vi "练习3.2-连续改变输出频率.vi"() -> ()   [LabVIEW 2021]
panel:
  out "Waveform Graph":dynamicdata(graph)
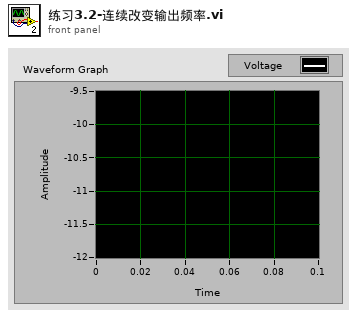
[diagram p1: front panel]
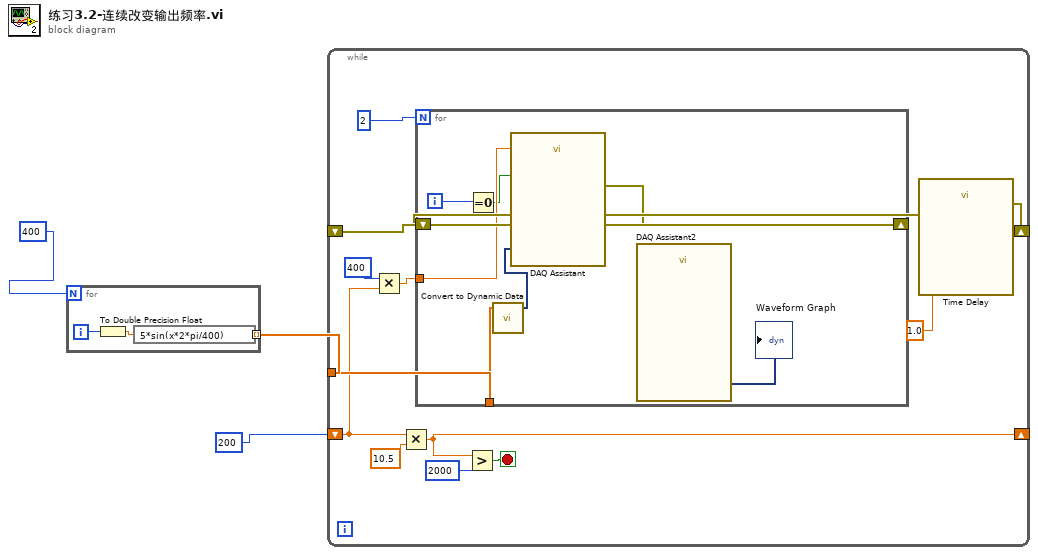
[diagram p0: block diagram]
diagram:
  n1 = for {
    N: 400 -> [_]
    tunnel: [w4] -> w3 mode=indexing
    i -> [w6]
    n2 = To Double Precision Float(number=w6) -> (double precision float=w5:dbl)
    n3 = expression code="5*sin(x*2*pi/400)"(w5) -> (w4:dbl)
  }
  n4 = while {
    tunnel: w3 -> [w18]
    shift-right: [w10] -> _
    shift-left: 200 -> [w14]
    shift-right: [w7] -> _
    shift-left: _ -> [w17]
    stop <- w11 stop-if-true
    n5 = Multiply(x=400, y=w14) -> (x*y=w15:dbl)
    n6 = Multiply(x=w14, y=10.5) -> (x*y=w10:dbl)
    n7 = for {
      N: 2 -> [_]
      tunnel: w18 -> [w25]
      shift-right: [w21] -> w8
      shift-left: w17 -> [_]
      tunnel: w15 -> [w24]
      i -> [w23]
      n8 = Equal To 0?(x=w23) -> (x = 0?=w22:bool)
      n9 = call "Convert to Dynamic Data"("Array"=w25) -> ("Dynamic Data Type"=w26:dynamicdata)  [unwired: 3 in]
      n10 = call "DAQ Assistant"("data"=w26, "rate"=w24, "stop (F)"=w22) -> ("error out"=w21:errorcluster)  [unwired: 14 in, 2 out]
      n11 = call "DAQ Assistant2"() -> ("data"=→"Waveform Graph":dynamicdata)  [unwired: 17 in, 2 out]
    }
    n12 = Greater?(x=w10, y=2000) -> (0:w11:bool)
    n13 = call "Time Delay"("error in (no error)"=w8, "Delay Time (s)"=1.0) -> ("error out"=w7:errorcluster)  [unwired: 9 in]
  }
